vi "setup Loop Frequency LV.vi"(10 "frequency":u16, 11 "instance":i32) -> (3 "function return":u32)   [LabVIEW 2023, in "SADI_FW3.lvlib"]
doc: "SADI_API_Wrapper unsigned int setupLoopFrequency_LV( int instance, uint16_t frequency );"
uses:
  SADI_FW3.lvlib
  SADI_FW3.dll
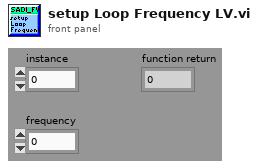
[diagram p1: front panel]
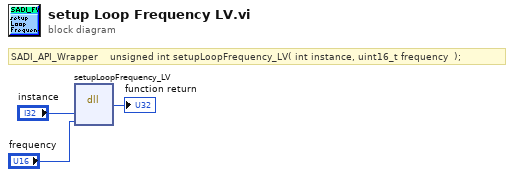
[diagram p0: block diagram]
diagram:
  # "SADI_API_Wrapper    unsigned int setupLoopFrequency_LV( int instance, uint16_t frequency  );"
  n1 = dll-call lib="C:/Users/loran/Documents/School/24_Spring/Controls Lab/EML4314c_Sp24_framework_0/LVLib/SADI_FW3.*" fn="setupLoopFrequency_LV"("instance"="instance", "frequency"="frequency") -> (→"function return":u32)  [unwired: 5 in, 2 out]
